vi "CmdConsole.Run and Wait single VI.vi"(6 "Workign Dir":path, 7 "IgnoreStdErr":bool, 8 "error in":errorcluster, 9 "Timeout":dbl, 10 "Args":string, 11 "App":path) -> (0 "error out":errorcluster, 1 "Duration(s)":dbl, 2 "Log":string, 3 "Output":string, 4 "RtnCode":i32)   [LabVIEW 2018]
uses:
  CmdConsole.lvclass
  <vilib>/KATE/Time/Time Utils.lvlib
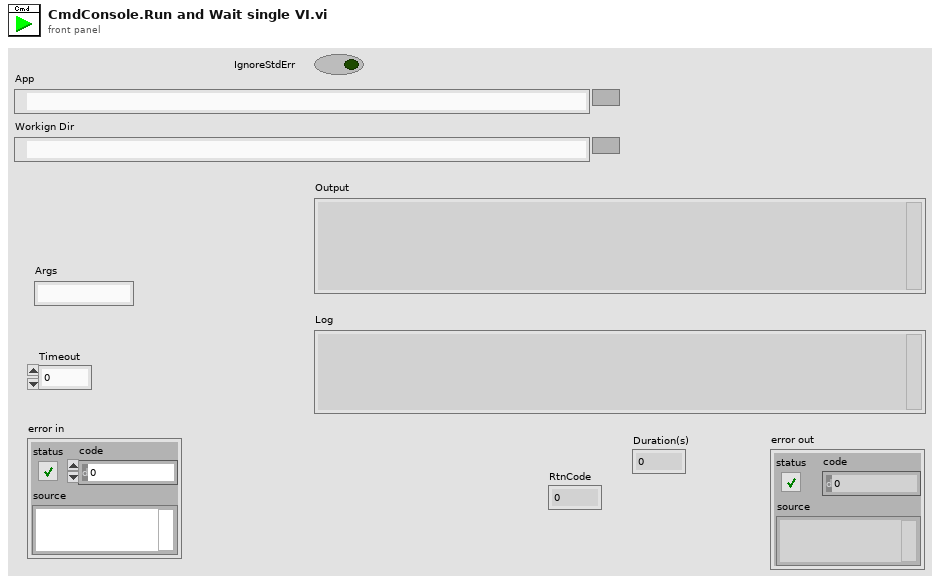
[diagram p1: front panel]
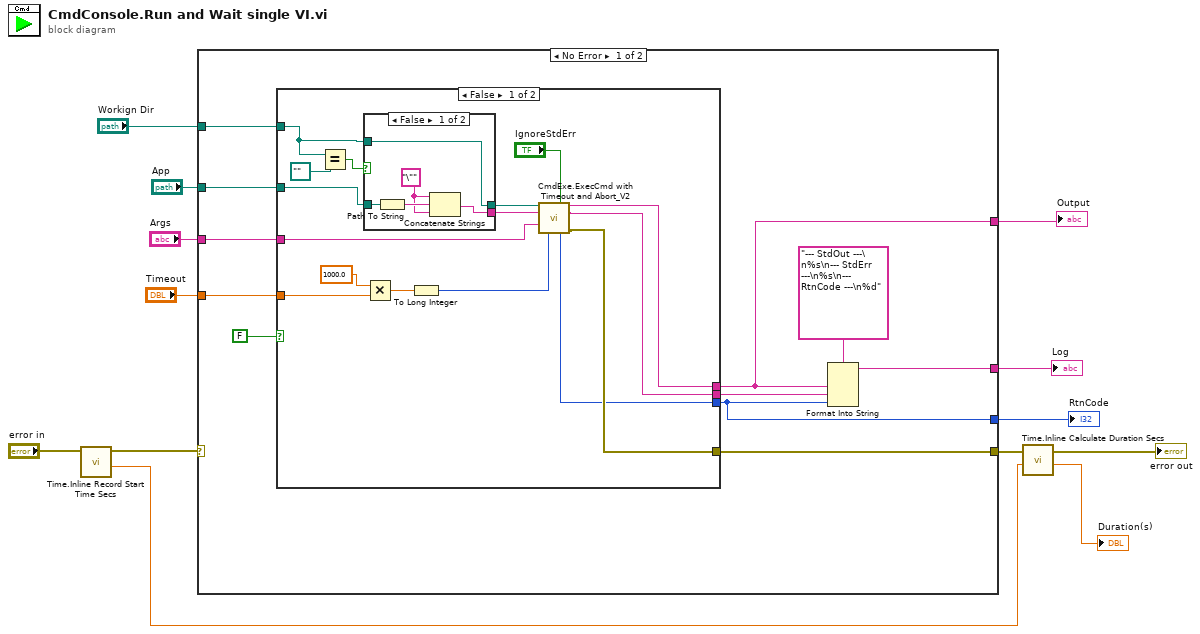
[diagram p0: block diagram]
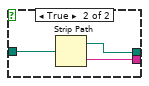
[diagram p2: hidden frame]
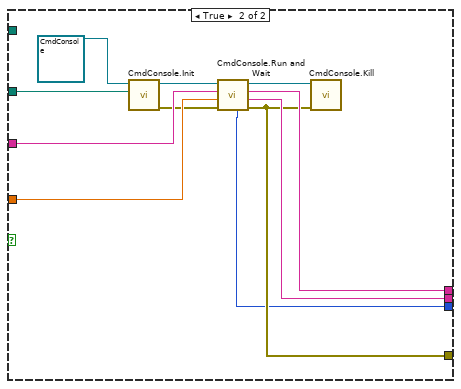
[diagram p3: hidden frame]
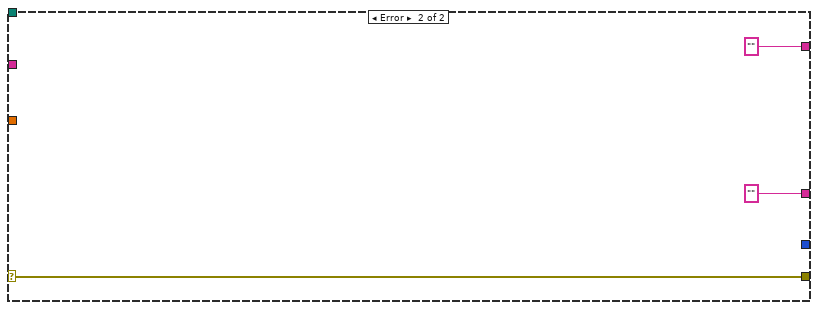
[diagram p4: hidden frame]
diagram:
  n1 = call <vilib>:"Time.Inline Record Start Time Secs.vi"("Error In Upper"="error in") -> ("Start(s)"=w4:dbl, "Error Out Upper"=w5:errorcluster)  [unwired: 8 in, 1 out]
  n2 = case shown="No Error" w5 {
    selector: w5 -> [_ w62]
    tunnel: "Timeout" -> [w24 _]
    tunnel: "App" -> [w23 _]
    tunnel: "Args" -> [w22 _]
    tunnel: [w19 ""] -> w10
    tunnel: [w18 "" ("Std Out")] -> w9
    tunnel: [w17 w62] -> w8
    tunnel: "Workign Dir" -> [w15 _]
    tunnel: [w14 _] -> w1
    frame No Error {
      n3 = case shown="False" FALSE {
        tunnel: w24 -> [w33 w57]
        tunnel: w23 -> [w40 w56]
        tunnel: w22 -> [w34 w55]
        tunnel: [w38 w53] -> w20
        tunnel: [w28 w50] -> w14
        tunnel: [w39 w52] -> w18
        tunnel: [w37 w51] -> w17
        tunnel: w15 -> [w25 _]
        frame False {
          n4 = Equal?(x=w25, y=path "") -> (x = y?=w27:bool)
          n5 = case shown="False" w27 {
            tunnel: w40 -> [w45 w48]
            tunnel: [w42 w47] -> w36
            tunnel: [w41 w46] -> w35
            tunnel: w25 -> [w42 _]
            frame False {
              w43 = "\""
              n6 = Path To String(path=w45) -> (string=w44:string)
              n7 = Concatenate Strings(w43, w44, w43) -> (w41:string)
            }
            frame True {
              n8 = Strip Path(path=w48) -> (stripped path=w47:path, name=w46:string)
            }
          }
          n9 = Multiply(x=1000.0, y=w33) -> (x*y=w31:dbl)
          n10 = To Long Integer(number=w31) -> (32bit integer=w30:i32)
          n11 = call "CmdExe.ExecCmd with Timeout and Abort_V2.vi"("Working Dir"=w36, "IgnoreStdErr"="IgnoreStdErr", "Executable"=w35, "Arguements"=w34, "Timeout ms(-1)"=w30) -> ("STD OUT"=w39:string, "STD ERR"=w38:string, "return code"=w28:i32, "error out"=w37:errorcluster)  [unwired: 5 in, 2 out]
        }
        frame True {
          n12 = call "CmdConsole.Init.vi"("App"=w56, "CmdConsole in"=refnum<class "CmdConsole.lvclass"> refnum) -> ("error out"=w54:errorcluster, "CmdConsole out"=w59:refnum<class "CmdConsole.lvclass">)  [unwired: 8 in]
          n13 = call "CmdConsole.Run and Wait.vi"("error in (no error)"=w54, "Timeout(s)"=w57, "Args"=w55, "CmdConsole in"=w59) -> ("error out"=w51:errorcluster, "Std Error"=w53:string, "Std Out"=w52:string, "CmdConsole out"=w58:refnum<class "CmdConsole.lvclass">, "RtnCode"=w50:i32)  [unwired: 2 in, 1 out]
          n14 = call "CmdConsole.Kill.vi"("error in"=w51, "CmdConsole in"=w58) -> ()  [unwired: 8 in, 2 out]
        }
      }
      n15 = Format Into String(format string="--- StdOut ---\n%s\n--- StdErr ---\n%s\n--- RtnCode ---\n%d", w18, w20, w14) -> (resulting string=w19:string)  [unwired: 2 in, 1 out]
    }
    frame Error {
    }
  }
  "Output" <- w9
  "Log" <- w10
  "RtnCode" <- w1
  n16 = call <vilib>:"Time.Inline Calculate Duration Secs.vi"("Start(Sec)"=w4, "Error In Top"=w8) -> ("Duration(s)"=→"Duration(s)":dbl, "Error Out Top"=→"error out":errorcluster)  [unwired: 7 in, 1 out]
